vi "InitializeMotorsXYZR.vi"(0 "COM PORT Array IN":refnum<visa-resource-name>[](array[refnum]), 1 "STEP SP Array IN":i32[](array[numeric]), 2 "XYZ in RANGE Array IN":bool[](array[boolean]), 3 "XYZR VEL PV Array IN":i32[](array[numeric]), 4 "RUNHOLDArray IN":i32[](array[numeric]), 5 "Error Array IN":errorcluster[](array[cluster])) -> (14 "COM PORT Array OUT":refnum<visa-resource-name>[](array[refnum]), 15 "STEP SP Array OUT":i32[](array[numeric]), 16 "XYZ in RANGE Array OUT":bool[](array[boolean]), 17 "XYZR VEL PV Array OUT":i32[](array[numeric]), 18 "XYZR MAX MIN POS":i32[](array[numeric]), 19 "Error Array OUT":errorcluster[](array[cluster]))   [LabVIEW 2009]
panel:
  out "R velocity PV step/sec[3]":i32
  out "Z velocity PV step/sec[2]":i32
  out "Y velocity PV step/sec[1]":i32
  out "X velocity PV step/sec[0]":i32
  out "R in Range[3]":bool
  out "Z in Range[2]":bool
  out "Y in Range[1]":bool
  out "X in Range[0]":bool
  out "R Step SP[3]":i32
  out "Z Step SP[2]":i32
  out "Y Step SP[1]":i32 min=-2304000 max=2304000
  out "X Velocity SP step/sec[4]":i32
  out "Y Velocity SP step/sec[5]":i32
  out "Z Velocity SP step/sec[6]":i32
  out "R Velocity SP step/sec[7]":i32
  out "X Step SP[0]":i32 min=-2304000 max=2304000
  out "Z Run Holding %[7]":i32
  out "R Run Current %[6]":i32
  out "R Run Holding %[5]":i32
  out "Y Run Current %[4]":i32
  out "Y Run Holding %[3]":i32
  out "Z Run Current %[2]":i32
  out "X Run Holding %[1]":i32
  out "X Run Current %[0]":i32
  out "X MINPOS":i32=-94296
  out "X MAXPOS":i32=-34296
  out "Y MINPOS":i32=-94296
  out "Y MAXPOS":i32=-34296
  out "R MAXPOS":i32=-34296
  out "R MINPOS":i32=-94296
  out "Z MINPOS":i32=-94296
  out "Z MAXPOS":i32=-34296
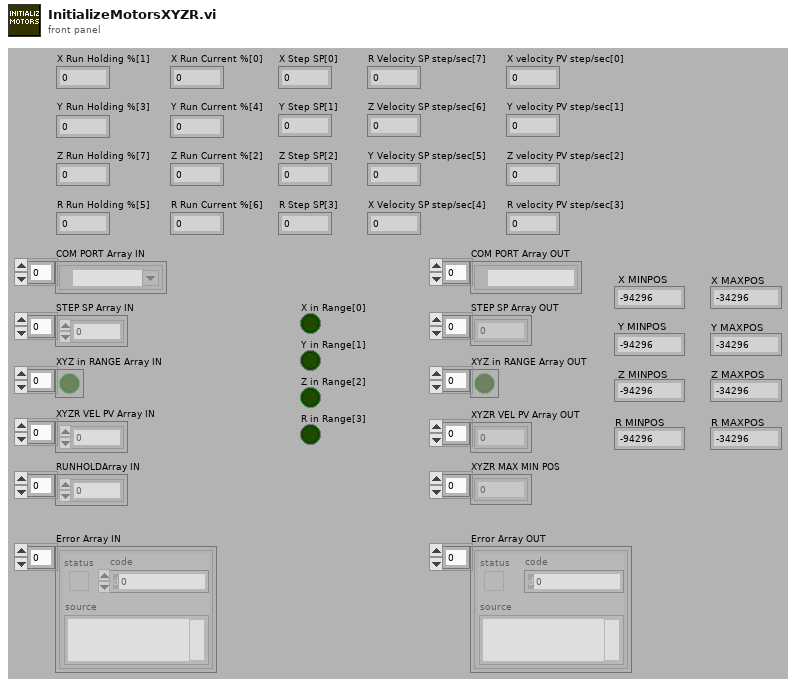
[diagram p1: front panel]
types:
  T1 = cluster{"XYZ in RANGE Array IN[0]":bool, "XYZ in RANGE Array IN[1]":bool, "XYZ in RANGE Array IN[2]":bool, "XYZ in RANGE Array IN[3]":bool, "XYZ in RANGE Array IN[4]":bool, "XYZ in RANGE Array IN[5]":bool, "XYZ in RANGE Array IN[6]":bool, "XYZ in RANGE Array IN[7]":bool, "XYZ in RANGE Array IN[8]":bool}
  T2 = cluster{"XYZR VEL PV Array IN[0]":i32, "XYZR VEL PV Array IN[1]":i32, "XYZR VEL PV Array IN[2]":i32, "XYZR VEL PV Array IN[3]":i32, "XYZR VEL PV Array IN[4]":i32, "XYZR VEL PV Array IN[5]":i32, "XYZR VEL PV Array IN[6]":i32, "XYZR VEL PV Array IN[7]":i32, "XYZR VEL PV Array IN[8]":i32}
  T3 = cluster{"COM PORT Array IN[0]":refnum<visa-resource-name>, "COM PORT Array IN[1]":refnum<visa-resource-name>, "COM PORT Array IN[2]":refnum<visa-resource-name>, "COM PORT Array IN[3]":refnum<visa-resource-name>, "COM PORT Array IN[4]":refnum<visa-resource-name>, "COM PORT Array IN[5]":refnum<visa-resource-name>, "COM PORT Array IN[6]":refnum<visa-resource-name>, "COM PORT Array IN[7]":refnum<visa-resource-name>, "COM PORT Array IN[8]":refnum<visa-resource-name>}
  T4 = cluster{"Error Array IN[0]":errorcluster, "Error Array IN[1]":errorcluster, "Error Array IN[2]":errorcluster, "Error Array IN[3]":errorcluster, "Error Array IN[4]":errorcluster, "Error Array IN[5]":errorcluster, "Error Array IN[6]":errorcluster, "Error Array IN[7]":errorcluster, "Error Array IN[8]":errorcluster}
  T5 = cluster{"RUNHOLDArray IN[0]":i32, "RUNHOLDArray IN[1]":i32, "RUNHOLDArray IN[2]":i32, "RUNHOLDArray IN[3]":i32, "RUNHOLDArray IN[4]":i32, "RUNHOLDArray IN[5]":i32, "RUNHOLDArray IN[6]":i32, "RUNHOLDArray IN[7]":i32, "RUNHOLDArray IN[8]":i32}
  T6 = cluster{"STEP SP Array IN[0]":i32, "STEP SP Array IN[1]":i32, "STEP SP Array IN[2]":i32, "STEP SP Array IN[3]":i32, "STEP SP Array IN[4]":i32, "STEP SP Array IN[5]":i32, "STEP SP Array IN[6]":i32, "STEP SP Array IN[7]":i32, "STEP SP Array IN[8]":i32}
  T7 = enum16{"Stop", "Reset", "Run Current", "Holding Current", "Accel Rate", "Decel Rate", "Move to Relative Position", "Move to Absolute Position", "Echo Mode", "Print Parameter", "Send String", "Microstep Resolution", "Set Current Position", "Max Velocity"}
  T8 = cluster{"VISA resource name out":refnum<visa-resource-name>, "VISA resource name out":refnum<visa-resource-name>, "VISA resource name out":refnum<visa-resource-name>, "VISA resource name out":refnum<visa-resource-name>}
  T9 = cluster{"error out":errorcluster, "error out":errorcluster, "error out":errorcluster, "error out":errorcluster}
  T10 = cluster{"Value":i32, "Value":i32, "Value":i32, "Value":i32, "Value":i32, "Value":i32, "Value":i32, "Value":i32}
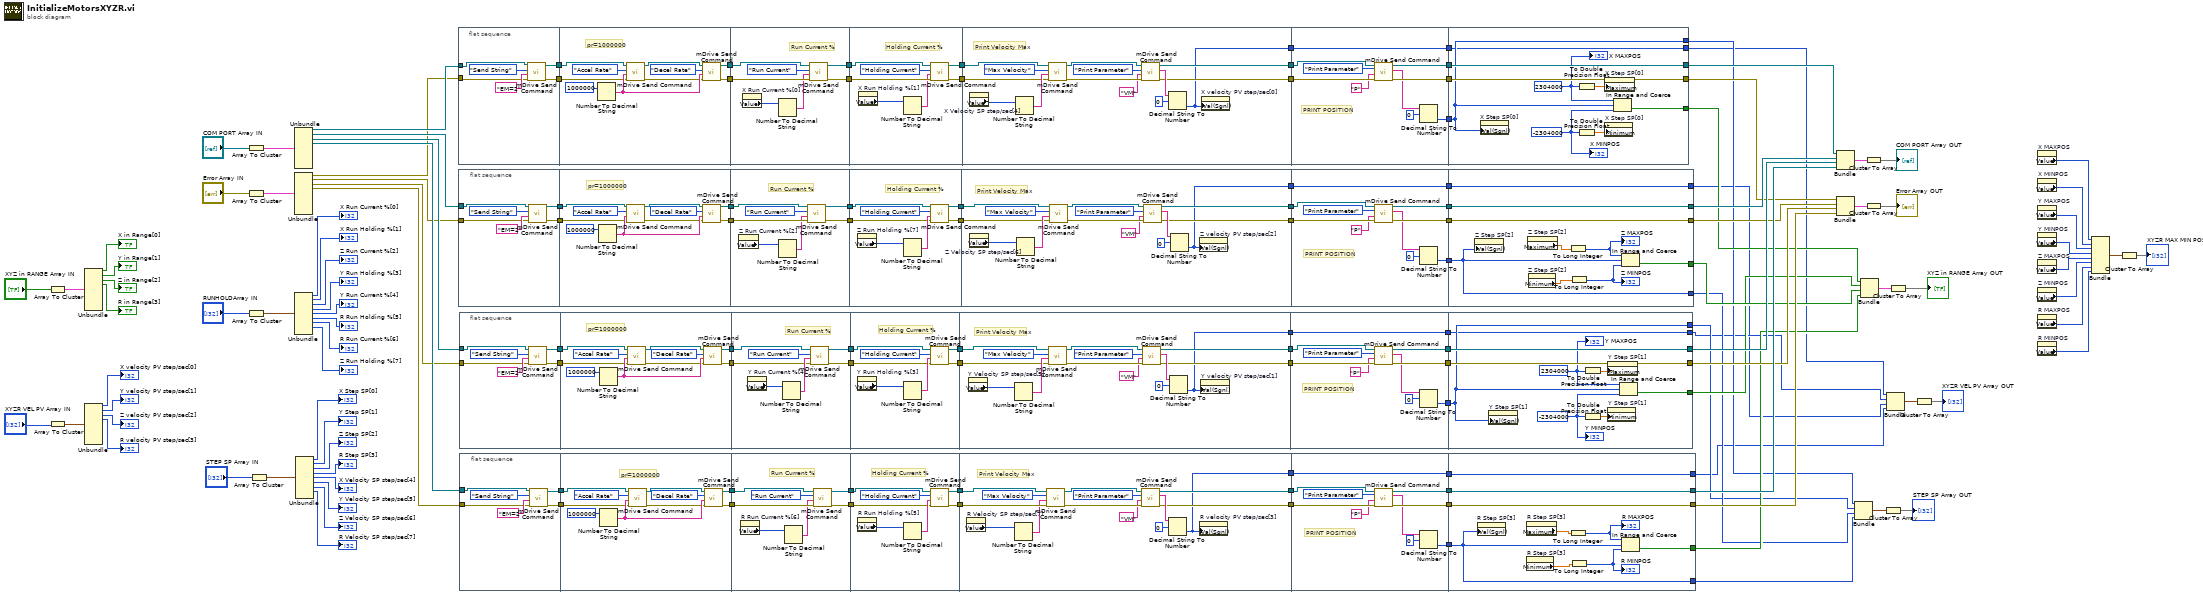
[diagram p0: block diagram]
diagram:
  n1 = Array To Cluster(array="XYZ in RANGE Array IN") -> (cluster=w55:T1)
  n2 = Array To Cluster(array="XYZR VEL PV Array IN") -> (cluster=w54:T2)
  n3 = Unbundle(w55) -> ("XYZ in RANGE Array IN[0]"=→"X in Range[0]":bool, "XYZ in RANGE Array IN[1]"=→"Y in Range[1]":bool, "XYZ in RANGE Array IN[2]"=→"Z in Range[2]":bool, "XYZ in RANGE Array IN[3]"=→"R in Range[3]":bool)  [unwired: 5 out]
  n4 = Unbundle(w54) -> ("XYZR VEL PV Array IN[0]"=→"X velocity PV step/sec[0]":i32, "XYZR VEL PV Array IN[1]"=→"Y velocity PV step/sec[1]":i32, "XYZR VEL PV Array IN[2]"=→"Z velocity PV step/sec[2]":i32, "XYZR VEL PV Array IN[3]"=→"R velocity PV step/sec[3]":i32)  [unwired: 5 out]
  n5 = Array To Cluster(array="COM PORT Array IN") -> (cluster=w90:T3)
  n6 = Array To Cluster(array="Error Array IN") -> (cluster=w89:T4)
  n7 = Array To Cluster(array="RUNHOLDArray IN") -> (cluster=w67:T5)
  n8 = Array To Cluster(array="STEP SP Array IN") -> (cluster=w53:T6)
  n9 = Unbundle(w90) -> ("COM PORT Array IN[0]"=w88:refnum<visa-resource-name>, "COM PORT Array IN[1]"=w87:refnum<visa-resource-name>, "COM PORT Array IN[2]"=w86:refnum<visa-resource-name>, "COM PORT Array IN[3]"=w85:refnum<visa-resource-name>)  [unwired: 5 out]
  n10 = Unbundle(w89) -> ("Error Array IN[0]"=w84:errorcluster, "Error Array IN[1]"=w83:errorcluster, "Error Array IN[2]"=w82:errorcluster, "Error Array IN[3]"=w81:errorcluster)  [unwired: 5 out]
  n11 = Unbundle(w67) -> ("RUNHOLDArray IN[0]"=→"X Run Current %[0]":i32, "RUNHOLDArray IN[1]"=→"X Run Holding %[1]":i32, "RUNHOLDArray IN[2]"=→"Z Run Current %[2]":i32, "RUNHOLDArray IN[3]"=→"Y Run Holding %[3]":i32, "RUNHOLDArray IN[4]"=→"Y Run Current %[4]":i32, "RUNHOLDArray IN[5]"=→"R Run Holding %[5]":i32, "RUNHOLDArray IN[6]"=→"R Run Current %[6]":i32, "RUNHOLDArray IN[7]"=→"Z Run Holding %[7]":i32)  [unwired: 1 out]
  n12 = Unbundle(w53) -> ("STEP SP Array IN[0]"=→"X Step SP[0]":i32, "STEP SP Array IN[1]"=→"Y Step SP[1]":i32, "STEP SP Array IN[2]"=→"Z Step SP[2]":i32, "STEP SP Array IN[3]"=→"R Step SP[3]":i32, "STEP SP Array IN[4]"=→"X Velocity SP step/sec[4]":i32, "STEP SP Array IN[5]"=→"Y Velocity SP step/sec[5]":i32, "STEP SP Array IN[6]"=→"Z Velocity SP step/sec[6]":i32, "STEP SP Array IN[7]"=→"R Velocity SP step/sec[7]":i32)  [unwired: 1 out]
  n13 = flat-sequence {
    tunnel: [w148] -> w105
    tunnel: [w147] -> w104
    tunnel: w88 -> [w146]
    tunnel: w84 -> [w145]
    tunnel: w105 -> [w160]
    tunnel: [w156] -> w103
    tunnel: w104 -> [w153]
    tunnel: [w151] -> w102
    tunnel: [w164] -> w101
    tunnel: [w166] -> w100
    tunnel: w103 -> [w165]
    tunnel: w102 -> [w167]
    tunnel: w101 -> [w174]
    tunnel: [w173] -> w99
    tunnel: w100 -> [w171]
    tunnel: [w172] -> w98
    tunnel: [w184] -> w97
    tunnel: [w185] -> w96
    tunnel: w99 -> [w183]
    tunnel: w98 -> [w177]
    tunnel: [w175] -> w9
    tunnel: w97 -> [w196]
    tunnel: w96 -> [w195]
    tunnel: [w198] -> w95
    tunnel: [w197] -> w94
    tunnel: [w192] -> w93
    tunnel: w9 -> [w189]
    tunnel: [w189] -> w8
    tunnel: [w206] -> w74
    tunnel: [w207] -> w80
    tunnel: w95 -> [w207]
    tunnel: w94 -> [w206]
    tunnel: w93 -> [w200]
    tunnel: [w201] -> w20
    tunnel: [w200] -> w14
    tunnel: w8 -> [w199]
    tunnel: [w199] -> w4
    frame #0 {
      n14 = call "mDrive Send Command.vi"("error in (no error)"=w145, "Extra"="EM=2", "Command"=T7."Send String", "VISA resource name"=w146) -> ("error out"=w147:errorcluster, "VISA resource name out"=w148:refnum<visa-resource-name>)  [unwired: 3 in, 1 out]
    }
    frame #1 {
      # "pr=1000000"
      n15 = Number To Decimal String(number=1000000) -> (decimal integer string=w154:string)  [unwired: 1 in]
      n16 = call "mDrive Send Command.vi"("error in (no error)"=w153, "Extra"=w154, "Command"=T7."Accel Rate", "VISA resource name"=w160) -> ("error out"=w152:errorcluster, "VISA resource name out"=w159:refnum<visa-resource-name>)  [unwired: 3 in, 1 out]
      n17 = call "mDrive Send Command.vi"("error in (no error)"=w152, "Extra"=w154, "Command"=T7."Decel Rate", "VISA resource name"=w159) -> ("error out"=w151:errorcluster, "VISA resource name out"=w156:refnum<visa-resource-name>)  [unwired: 3 in, 1 out]
    }
    frame #2 {
      # "Run Current %"
      n18 = property on="X Run Current %[0]" class="DigNum (strict)"() -> ("Value"=w161:i32)  [unwired: 2 in, 2 out]
      n19 = Number To Decimal String(number=w161) -> (decimal integer string=w163:string)  [unwired: 1 in]
      n20 = call "mDrive Send Command.vi"("error in (no error)"=w167, "Extra"=w163, "Command"=T7."Run Current", "VISA resource name"=w165) -> ("error out"=w166:errorcluster, "VISA resource name out"=w164:refnum<visa-resource-name>)  [unwired: 3 in, 1 out]
    }
    frame #3 {
      # "Holding Current %"
      n21 = property on="X Run Holding %[1]" class="DigNum (strict)"() -> ("Value"=w168:i32)  [unwired: 2 in, 2 out]
      n22 = Number To Decimal String(number=w168) -> (decimal integer string=w170:string)  [unwired: 1 in]
      n23 = call "mDrive Send Command.vi"("error in (no error)"=w171, "Extra"=w170, "Command"=T7."Holding Current", "VISA resource name"=w174) -> ("error out"=w172:errorcluster, "VISA resource name out"=w173:refnum<visa-resource-name>)  [unwired: 3 in, 1 out]
    }
    frame #4 {
      # "Print Velocity Max"
      n24 = property on="X Velocity SP step/sec[4]" class="DigNum (strict)"() -> ("Value"=w176:i32)  [unwired: 2 in, 2 out]
      n25 = Number To Decimal String(number=w176) -> (decimal integer string=w182:string)  [unwired: 1 in]
      n26 = call "mDrive Send Command.vi"("error in (no error)"=w177, "Extra"=w182, "Command"=T7."Max Velocity", "VISA resource name"=w183) -> ("error out"=w181:errorcluster, "VISA resource name out"=w188:refnum<visa-resource-name>)  [unwired: 3 in, 1 out]
      n27 = call "mDrive Send Command.vi"("error in (no error)"=w181, "Extra"="VM", "Command"=T7."Print Parameter", "VISA resource name"=w188) -> ("error out"=w185:errorcluster, "read buffer"=w186:string, "VISA resource name out"=w184:refnum<visa-resource-name>)  [unwired: 3 in]
      n28 = Decimal String To Number(string=w186, offset=0) -> (number=w175:i32)  [unwired: 1 in, 1 out]
      n29 = property on="X velocity PV step/sec[0]" class="DigNum (strict)"("Val(Sgnl)"=w175) -> ()  [unwired: 2 in, 2 out]
    }
    frame #5 {
      # "PRINT POSITION"
      n30 = call "mDrive Send Command.vi"("error in (no error)"=w195, "Extra"="P", "Command"=T7."Print Parameter", "VISA resource name"=w196) -> ("error out"=w197:errorcluster, "read buffer"=w194:string, "VISA resource name out"=w198:refnum<visa-resource-name>)  [unwired: 3 in]
      n31 = Decimal String To Number(string=w194, offset=0) -> (number=w192:i32)  [unwired: 1 in, 1 out]
    }
    frame #6 {
      w205 = -2304000 ("lower limit")
      w204 = 2304000 ("upper limit")
      n32 = property on="X Step SP[0]" class="DigNum (strict)"("Val(Sgnl)"=w200) -> ()  [unwired: 2 in, 2 out]
      n33 = To Double Precision Float(number=w204) -> (double precision float=w203:dbl)
      n34 = To Double Precision Float(number=w205) -> (double precision float=w202:dbl)
      n35 = property on="X Step SP[0]" class="DigNum (strict)"("Maximum"=w203) -> ()  [unwired: 2 in, 2 out]
      n36 = property on="X Step SP[0]" class="DigNum (strict)"("Minimum"=w202) -> ()  [unwired: 2 in, 2 out]
      n37 = In Range and Coerce(upper limit=w204, x=w200, lower limit=w205) -> (In Range?=w201:bool)  [unwired: 1 out]
      "X MINPOS" <- w205
      "X MAXPOS" <- w204
    }
  }
  n38 = flat-sequence {
    tunnel: [w211] -> w144
    tunnel: [w210] -> w143
    tunnel: w87 -> [w209]
    tunnel: w83 -> [w208]
    tunnel: w144 -> [w223]
    tunnel: [w219] -> w142
    tunnel: w143 -> [w216]
    tunnel: [w214] -> w141
    tunnel: [w227] -> w140
    tunnel: [w229] -> w139
    tunnel: w142 -> [w228]
    tunnel: w141 -> [w230]
    tunnel: w140 -> [w237]
    tunnel: [w236] -> w138
    tunnel: w139 -> [w232]
    tunnel: [w235] -> w137
    tunnel: [w247] -> w136
    tunnel: [w248] -> w135
    tunnel: w138 -> [w246]
    tunnel: w137 -> [w240]
    tunnel: [w238] -> w10
    tunnel: w136 -> [w259]
    tunnel: w135 -> [w258]
    tunnel: [w261] -> w134
    tunnel: [w260] -> w133
    tunnel: [w255] -> w132
    tunnel: w10 -> [w252]
    tunnel: [w252] -> w7
    tunnel: [w269] -> w73
    tunnel: [w270] -> w79
    tunnel: w134 -> [w270]
    tunnel: w133 -> [w269]
    tunnel: w132 -> [w263]
    tunnel: [w264] -> w19
    tunnel: [w263] -> w15
    tunnel: w7 -> [w262]
    tunnel: [w262] -> w2
    frame #0 {
      n39 = call "mDrive Send Command.vi"("error in (no error)"=w208, "Extra"="EM=2", "Command"=T7."Send String", "VISA resource name"=w209) -> ("error out"=w210:errorcluster, "VISA resource name out"=w211:refnum<visa-resource-name>)  [unwired: 3 in, 1 out]
    }
    frame #1 {
      # "pr=1000000"
      n40 = Number To Decimal String(number=1000000) -> (decimal integer string=w217:string)  [unwired: 1 in]
      n41 = call "mDrive Send Command.vi"("error in (no error)"=w216, "Extra"=w217, "Command"=T7."Accel Rate", "VISA resource name"=w223) -> ("error out"=w215:errorcluster, "VISA resource name out"=w222:refnum<visa-resource-name>)  [unwired: 3 in, 1 out]
      n42 = call "mDrive Send Command.vi"("error in (no error)"=w215, "Extra"=w217, "Command"=T7."Decel Rate", "VISA resource name"=w222) -> ("error out"=w214:errorcluster, "VISA resource name out"=w219:refnum<visa-resource-name>)  [unwired: 3 in, 1 out]
    }
    frame #2 {
      # "Run Current %"
      n43 = property on="Z Run Current %[2]" class="DigNum (strict)"() -> ("Value"=w224:i32)  [unwired: 2 in, 2 out]
      n44 = Number To Decimal String(number=w224) -> (decimal integer string=w226:string)  [unwired: 1 in]
      n45 = call "mDrive Send Command.vi"("error in (no error)"=w230, "Extra"=w226, "Command"=T7."Run Current", "VISA resource name"=w228) -> ("error out"=w229:errorcluster, "VISA resource name out"=w227:refnum<visa-resource-name>)  [unwired: 3 in, 1 out]
    }
    frame #3 {
      # "Holding Current %"
      n46 = property on="Z Run Holding %[7]" class="DigNum (strict)"() -> ("Value"=w231:i32)  [unwired: 2 in, 2 out]
      n47 = Number To Decimal String(number=w231) -> (decimal integer string=w234:string)  [unwired: 1 in]
      n48 = call "mDrive Send Command.vi"("error in (no error)"=w232, "Extra"=w234, "Command"=T7."Holding Current", "VISA resource name"=w237) -> ("error out"=w235:errorcluster, "VISA resource name out"=w236:refnum<visa-resource-name>)  [unwired: 3 in, 1 out]
    }
    frame #4 {
      # "Print Velocity Max"
      n49 = property on="Z Velocity SP step/sec[6]" class="DigNum (strict)"() -> ("Value"=w239:i32)  [unwired: 2 in, 2 out]
      n50 = Number To Decimal String(number=w239) -> (decimal integer string=w245:string)  [unwired: 1 in]
      n51 = call "mDrive Send Command.vi"("error in (no error)"=w240, "Extra"=w245, "Command"=T7."Max Velocity", "VISA resource name"=w246) -> ("error out"=w244:errorcluster, "VISA resource name out"=w251:refnum<visa-resource-name>)  [unwired: 3 in, 1 out]
      n52 = call "mDrive Send Command.vi"("error in (no error)"=w244, "Extra"="VM", "Command"=T7."Print Parameter", "VISA resource name"=w251) -> ("error out"=w248:errorcluster, "read buffer"=w249:string, "VISA resource name out"=w247:refnum<visa-resource-name>)  [unwired: 3 in]
      n53 = Decimal String To Number(string=w249, offset=0) -> (number=w238:i32)  [unwired: 1 in, 1 out]
      n54 = property on="Z velocity PV step/sec[2]" class="DigNum (strict)"("Val(Sgnl)"=w238) -> ()  [unwired: 2 in, 2 out]
    }
    frame #5 {
      # "PRINT POSITION"
      n55 = call "mDrive Send Command.vi"("error in (no error)"=w258, "Extra"="P", "Command"=T7."Print Parameter", "VISA resource name"=w259) -> ("error out"=w260:errorcluster, "read buffer"=w257:string, "VISA resource name out"=w261:refnum<visa-resource-name>)  [unwired: 3 in]
      n56 = Decimal String To Number(string=w257, offset=0) -> (number=w255:i32)  [unwired: 1 in, 1 out]
    }
    frame #6 {
      n57 = property on="Z Step SP[2]" class="DigNum (strict)"("Val(Sgnl)"=w263) -> ()  [unwired: 2 in, 2 out]
      n58 = property on="Z Step SP[2]" class="DigNum (strict)"() -> ("Maximum"=w266:dbl)  [unwired: 2 in, 2 out]
      n59 = property on="Z Step SP[2]" class="DigNum (strict)"() -> ("Minimum"=w265:dbl)  [unwired: 2 in, 2 out]
      n60 = To Long Integer(number=w266) -> (32bit integer=w268:i32)
      "Z MAXPOS" <- w268
      n61 = To Long Integer(number=w265) -> (32bit integer=w267:i32)
      "Z MINPOS" <- w267
      n62 = In Range and Coerce(upper limit=w268, x=w263, lower limit=w267) -> (In Range?=w264:bool)  [unwired: 1 out]
    }
  }
  n63 = flat-sequence {
    tunnel: [w274] -> w118
    tunnel: [w273] -> w117
    tunnel: w86 -> [w272]
    tunnel: w82 -> [w271]
    tunnel: w118 -> [w286]
    tunnel: [w282] -> w116
    tunnel: w117 -> [w279]
    tunnel: [w277] -> w115
    tunnel: [w291] -> w114
    tunnel: [w293] -> w113
    tunnel: w116 -> [w292]
    tunnel: w115 -> [w288]
    tunnel: w114 -> [w300]
    tunnel: [w299] -> w112
    tunnel: w113 -> [w295]
    tunnel: [w298] -> w111
    tunnel: [w310] -> w110
    tunnel: [w311] -> w109
    tunnel: w112 -> [w309]
    tunnel: w111 -> [w303]
    tunnel: [w301] -> w11
    tunnel: w110 -> [w322]
    tunnel: w109 -> [w321]
    tunnel: [w324] -> w108
    tunnel: [w323] -> w107
    tunnel: [w318] -> w106
    tunnel: w11 -> [w315]
    tunnel: [w315] -> w6
    tunnel: [w332] -> w72
    tunnel: [w333] -> w78
    tunnel: w108 -> [w333]
    tunnel: w107 -> [w332]
    tunnel: w106 -> [w326]
    tunnel: [w327] -> w18
    tunnel: [w326] -> w13
    tunnel: w6 -> [w325]
    tunnel: [w325] -> w3
    frame #0 {
      n64 = call "mDrive Send Command.vi"("error in (no error)"=w271, "Extra"="EM=2", "Command"=T7."Send String", "VISA resource name"=w272) -> ("error out"=w273:errorcluster, "VISA resource name out"=w274:refnum<visa-resource-name>)  [unwired: 3 in, 1 out]
    }
    frame #1 {
      # "pr=1000000"
      n65 = Number To Decimal String(number=1000000) -> (decimal integer string=w280:string)  [unwired: 1 in]
      n66 = call "mDrive Send Command.vi"("error in (no error)"=w279, "Extra"=w280, "Command"=T7."Accel Rate", "VISA resource name"=w286) -> ("error out"=w278:errorcluster, "VISA resource name out"=w285:refnum<visa-resource-name>)  [unwired: 3 in, 1 out]
      n67 = call "mDrive Send Command.vi"("error in (no error)"=w278, "Extra"=w280, "Command"=T7."Decel Rate", "VISA resource name"=w285) -> ("error out"=w277:errorcluster, "VISA resource name out"=w282:refnum<visa-resource-name>)  [unwired: 3 in, 1 out]
    }
    frame #2 {
      # "Run Current %"
      n68 = property on="Y Run Current %[4]" class="DigNum (strict)"() -> ("Value"=w287:i32)  [unwired: 2 in, 2 out]
      n69 = Number To Decimal String(number=w287) -> (decimal integer string=w290:string)  [unwired: 1 in]
      n70 = call "mDrive Send Command.vi"("error in (no error)"=w288, "Extra"=w290, "Command"=T7."Run Current", "VISA resource name"=w292) -> ("error out"=w293:errorcluster, "VISA resource name out"=w291:refnum<visa-resource-name>)  [unwired: 3 in, 1 out]
    }
    frame #3 {
      # "Holding Current %"
      n71 = property on="Y Run Holding %[3]" class="DigNum (strict)"() -> ("Value"=w294:i32)  [unwired: 2 in, 2 out]
      n72 = Number To Decimal String(number=w294) -> (decimal integer string=w297:string)  [unwired: 1 in]
      n73 = call "mDrive Send Command.vi"("error in (no error)"=w295, "Extra"=w297, "Command"=T7."Holding Current", "VISA resource name"=w300) -> ("error out"=w298:errorcluster, "VISA resource name out"=w299:refnum<visa-resource-name>)  [unwired: 3 in, 1 out]
    }
    frame #4 {
      # "Print Velocity Max"
      n74 = property on="Y Velocity SP step/sec[5]" class="DigNum (strict)"() -> ("Value"=w302:i32)  [unwired: 2 in, 2 out]
      n75 = Number To Decimal String(number=w302) -> (decimal integer string=w308:string)  [unwired: 1 in]
      n76 = call "mDrive Send Command.vi"("error in (no error)"=w303, "Extra"=w308, "Command"=T7."Max Velocity", "VISA resource name"=w309) -> ("error out"=w307:errorcluster, "VISA resource name out"=w314:refnum<visa-resource-name>)  [unwired: 3 in, 1 out]
      n77 = call "mDrive Send Command.vi"("error in (no error)"=w307, "Extra"="VM", "Command"=T7."Print Parameter", "VISA resource name"=w314) -> ("error out"=w311:errorcluster, "read buffer"=w312:string, "VISA resource name out"=w310:refnum<visa-resource-name>)  [unwired: 3 in]
      n78 = Decimal String To Number(string=w312, offset=0) -> (number=w301:i32)  [unwired: 1 in, 1 out]
      n79 = property on="Y velocity PV step/sec[1]" class="DigNum (strict)"("Val(Sgnl)"=w301) -> ()  [unwired: 2 in, 2 out]
    }
    frame #5 {
      # "PRINT POSITION"
      n80 = call "mDrive Send Command.vi"("error in (no error)"=w321, "Extra"="P", "Command"=T7."Print Parameter", "VISA resource name"=w322) -> ("error out"=w323:errorcluster, "read buffer"=w320:string, "VISA resource name out"=w324:refnum<visa-resource-name>)  [unwired: 3 in]
      n81 = Decimal String To Number(string=w320, offset=0) -> (number=w318:i32)  [unwired: 1 in, 1 out]
    }
    frame #6 {
      w330 = -2304000 ("lower limit")
      w331 = 2304000 ("upper limit")
      n82 = property on="Y Step SP[1]" class="DigNum (strict)"("Val(Sgnl)"=w326) -> ()  [unwired: 2 in, 2 out]
      n83 = To Double Precision Float(number=w331) -> (double precision float=w329:dbl)
      n84 = To Double Precision Float(number=w330) -> (double precision float=w328:dbl)
      n85 = property on="Y Step SP[1]" class="DigNum (strict)"("Maximum"=w329) -> ()  [unwired: 2 in, 2 out]
      n86 = property on="Y Step SP[1]" class="DigNum (strict)"("Minimum"=w328) -> ()  [unwired: 2 in, 2 out]
      n87 = In Range and Coerce(upper limit=w331, x=w326, lower limit=w330) -> (In Range?=w327:bool)  [unwired: 1 out]
      "Y MINPOS" <- w330
      "Y MAXPOS" <- w331
    }
  }
  n88 = flat-sequence {
    tunnel: [w337] -> w131
    tunnel: [w336] -> w130
    tunnel: w85 -> [w335]
    tunnel: w81 -> [w334]
    tunnel: w131 -> [w349]
    tunnel: [w345] -> w129
    tunnel: w130 -> [w342]
    tunnel: [w340] -> w128
    tunnel: [w353] -> w127
    tunnel: [w355] -> w126
    tunnel: w129 -> [w354]
    tunnel: w128 -> [w356]
    tunnel: w127 -> [w363]
    tunnel: [w362] -> w125
    tunnel: w126 -> [w358]
    tunnel: [w361] -> w124
    tunnel: [w373] -> w123
    tunnel: [w374] -> w122
    tunnel: w125 -> [w372]
    tunnel: w124 -> [w371]
    tunnel: [w364] -> w12
    tunnel: w123 -> [w385]
    tunnel: w122 -> [w384]
    tunnel: [w387] -> w121
    tunnel: [w386] -> w120
    tunnel: [w381] -> w119
    tunnel: w12 -> [w378]
    tunnel: [w378] -> w5
    tunnel: [w395] -> w71
    tunnel: [w396] -> w77
    tunnel: w121 -> [w396]
    tunnel: w120 -> [w395]
    tunnel: w119 -> [w389]
    tunnel: [w390] -> w17
    tunnel: [w389] -> w16
    tunnel: w5 -> [w388]
    tunnel: [w388] -> w1
    frame #0 {
      n89 = call "mDrive Send Command.vi"("error in (no error)"=w334, "Extra"="EM=2", "Command"=T7."Send String", "VISA resource name"=w335) -> ("error out"=w336:errorcluster, "VISA resource name out"=w337:refnum<visa-resource-name>)  [unwired: 3 in, 1 out]
    }
    frame #1 {
      # "pr=1000000"
      n90 = Number To Decimal String(number=1000000) -> (decimal integer string=w343:string)  [unwired: 1 in]
      n91 = call "mDrive Send Command.vi"("error in (no error)"=w342, "Extra"=w343, "Command"=T7."Accel Rate", "VISA resource name"=w349) -> ("error out"=w341:errorcluster, "VISA resource name out"=w348:refnum<visa-resource-name>)  [unwired: 3 in, 1 out]
      n92 = call "mDrive Send Command.vi"("error in (no error)"=w341, "Extra"=w343, "Command"=T7."Decel Rate", "VISA resource name"=w348) -> ("error out"=w340:errorcluster, "VISA resource name out"=w345:refnum<visa-resource-name>)  [unwired: 3 in, 1 out]
    }
    frame #2 {
      # "Run Current %"
      n93 = property on="R Run Current %[6]" class="DigNum (strict)"() -> ("Value"=w350:i32)  [unwired: 2 in, 2 out]
      n94 = Number To Decimal String(number=w350) -> (decimal integer string=w352:string)  [unwired: 1 in]
      n95 = call "mDrive Send Command.vi"("error in (no error)"=w356, "Extra"=w352, "Command"=T7."Run Current", "VISA resource name"=w354) -> ("error out"=w355:errorcluster, "VISA resource name out"=w353:refnum<visa-resource-name>)  [unwired: 3 in, 1 out]
    }
    frame #3 {
      # "Holding Current %"
      n96 = property on="R Run Holding %[5]" class="DigNum (strict)"() -> ("Value"=w357:i32)  [unwired: 2 in, 2 out]
      n97 = Number To Decimal String(number=w357) -> (decimal integer string=w360:string)  [unwired: 1 in]
      n98 = call "mDrive Send Command.vi"("error in (no error)"=w358, "Extra"=w360, "Command"=T7."Holding Current", "VISA resource name"=w363) -> ("error out"=w361:errorcluster, "VISA resource name out"=w362:refnum<visa-resource-name>)  [unwired: 3 in, 1 out]
    }
    frame #4 {
      # "Print Velocity Max"
      n99 = property on="R Velocity SP step/sec[7]" class="DigNum (strict)"() -> ("Value"=w365:i32)  [unwired: 2 in, 2 out]
      n100 = Number To Decimal String(number=w365) -> (decimal integer string=w370:string)  [unwired: 1 in]
      n101 = call "mDrive Send Command.vi"("error in (no error)"=w371, "Extra"=w370, "Command"=T7."Max Velocity", "VISA resource name"=w372) -> ("error out"=w369:errorcluster, "VISA resource name out"=w377:refnum<visa-resource-name>)  [unwired: 3 in, 1 out]
      n102 = call "mDrive Send Command.vi"("error in (no error)"=w369, "Extra"="VM", "Command"=T7."Print Parameter", "VISA resource name"=w377) -> ("error out"=w374:errorcluster, "read buffer"=w375:string, "VISA resource name out"=w373:refnum<visa-resource-name>)  [unwired: 3 in]
      n103 = Decimal String To Number(string=w375, offset=0) -> (number=w364:i32)  [unwired: 1 in, 1 out]
      n104 = property on="R velocity PV step/sec[3]" class="DigNum (strict)"("Val(Sgnl)"=w364) -> ()  [unwired: 2 in, 2 out]
    }
    frame #5 {
      # "PRINT POSITION"
      n105 = call "mDrive Send Command.vi"("error in (no error)"=w384, "Extra"="P", "Command"=T7."Print Parameter", "VISA resource name"=w385) -> ("error out"=w386:errorcluster, "read buffer"=w383:string, "VISA resource name out"=w387:refnum<visa-resource-name>)  [unwired: 3 in]
      n106 = Decimal String To Number(string=w383, offset=0) -> (number=w381:i32)  [unwired: 1 in, 1 out]
    }
    frame #6 {
      n107 = property on="R Step SP[3]" class="DigNum (strict)"("Val(Sgnl)"=w389) -> ()  [unwired: 2 in, 2 out]
      n108 = property on="R Step SP[3]" class="DigNum (strict)"() -> ("Maximum"=w391:dbl)  [unwired: 2 in, 2 out]
      n109 = property on="R Step SP[3]" class="DigNum (strict)"() -> ("Minimum"=w392:dbl)  [unwired: 2 in, 2 out]
      n110 = To Long Integer(number=w391) -> (32bit integer=w394:i32)
      "R MAXPOS" <- w394
      n111 = To Long Integer(number=w392) -> (32bit integer=w393:i32)
      "R MINPOS" <- w393
      n112 = In Range and Coerce(upper limit=w394, x=w389, lower limit=w393) -> (In Range?=w390:bool)  [unwired: 1 out]
    }
  }
  n113 = Bundle("VISA resource name out"=w80, "VISA resource name out"=w79, "VISA resource name out"=w78, "VISA resource name out"=w77) -> (w76:T8)  [unwired: 1 in]
  n114 = Bundle("error out"=w74, "error out"=w73, "error out"=w72, "error out"=w71) -> (w70:T9)  [unwired: 1 in]
  n115 = Bundle(w14, w13, w15, w16) -> (w32:cluster{i32, i32, i32, i32})  [unwired: 1 in]
  n116 = Bundle(w20, w18, w19, w17) -> (w36:cluster{bool, bool, bool, bool})  [unwired: 1 in]
  n117 = Cluster To Array(cluster=w76) -> (array=→"COM PORT Array OUT":refnum<visa-resource-name>[])
  n118 = Cluster To Array(cluster=w70) -> (array=→"Error Array OUT":errorcluster[])
  n119 = Cluster To Array(cluster=w32) -> (array=→"STEP SP Array OUT":i32[])
  n120 = Bundle(w4, w3, w2, w1) -> (w34:cluster{i32, i32, i32, i32})  [unwired: 1 in]
  n121 = Cluster To Array(cluster=w36) -> (array=→"XYZ in RANGE Array OUT":bool[])
  n122 = Cluster To Array(cluster=w34) -> (array=→"XYZR VEL PV Array OUT":i32[])
  n123 = property on="X MAXPOS" class="DigNum (strict)"() -> ("Value"=w29:i32)  [unwired: 2 in, 2 out]
  n124 = property on="X MINPOS" class="DigNum (strict)"() -> ("Value"=w23:i32)  [unwired: 2 in, 2 out]
  n125 = property on="Y MAXPOS" class="DigNum (strict)"() -> ("Value"=w22:i32)  [unwired: 2 in, 2 out]
  n126 = property on="Y MINPOS" class="DigNum (strict)"() -> ("Value"=w24:i32)  [unwired: 2 in, 2 out]
  n127 = property on="Z MAXPOS" class="DigNum (strict)"() -> ("Value"=w25:i32)  [unwired: 2 in, 2 out]
  n128 = property on="Z MINPOS" class="DigNum (strict)"() -> ("Value"=w26:i32)  [unwired: 2 in, 2 out]
  n129 = property on="R MAXPOS" class="DigNum (strict)"() -> ("Value"=w27:i32)  [unwired: 2 in, 2 out]
  n130 = property on="R MINPOS" class="DigNum (strict)"() -> ("Value"=w28:i32)  [unwired: 2 in, 2 out]
  n131 = Bundle("Value"=w29, "Value"=w23, "Value"=w22, "Value"=w24, "Value"=w25, "Value"=w26, "Value"=w27, "Value"=w28) -> (w30:T10)  [unwired: 1 in]
  n132 = Cluster To Array(cluster=w30) -> (array=→"XYZR MAX MIN POS":i32[])
